vi "Temperature measurement system.vi"() -> ()   [LabVIEW 2022 SP3]
panel:
  in  "stop":bool
  out "Voltage 2":dbl
  out "Voltage 1":dbl
  out "Resistance":dbl
  in  "R2":dbl
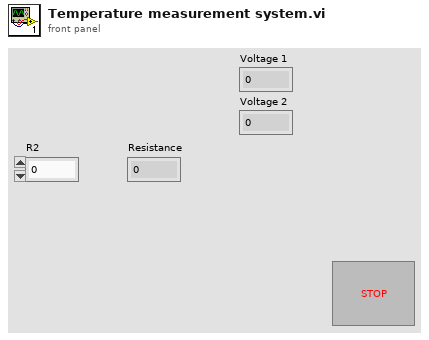
[diagram p1: front panel]
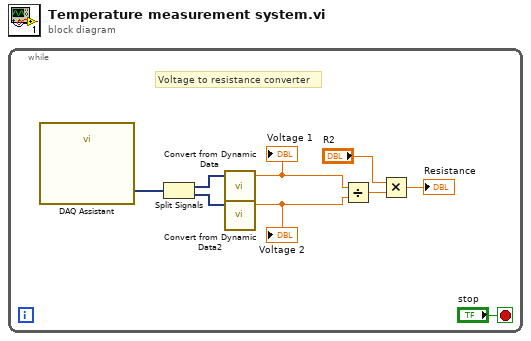
[diagram p0: block diagram]
diagram:
  n1 = while {
    stop <- "stop" stop-if-true
    # "Voltage to resistance converter"
    n2 = call "DAQ Assistant"() -> ("data"=w9:dynamicdata)  [unwired: 17 in, 2 out]
    n3 = Split Signals(w9) -> (w8:dynamicdata, w7:dynamicdata)  [unwired: 2 in]
    n4 = call "Convert from Dynamic Data"("Dynamic Data Type"=w8) -> ("Scalar"=w6:dbl)  [unwired: 3 in]
    "Voltage 1" <- w6
    n5 = call "Convert from Dynamic Data2"("Dynamic Data Type"=w7) -> ("Scalar"=w5:dbl)  [unwired: 3 in]
    "Voltage 2" <- w5
    n6 = Divide(x=w6, y=w5) -> (x/y=w3:dbl)
    n7 = Multiply(x="R2", y=w3) -> (x*y=→"Resistance":dbl)
  }
